vi "Object Items (poly).vi"   [LabVIEW 2019, in "JSONtext.lvlib"]
doc: "Find multiple Items in a JSON Object, by item names. Output items (as JSON) are in the same order as the supplied item names. If an item is not present, then the output for that item will be an empty string.\n\nThe location, in the input JSON, of the Object containing the items may be specified either by Offset or by a JSON Path (polymorphic input)."
uses:
  JSONtext.lvlib
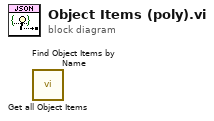
[diagram p0: block diagram]
diagram:
  n1 = call "Get all Object Items.vi"() -> ()  [unwired: 8 in, 4 out]
  n2 = call "Find Object Items by Name.vi"() -> ()  [unwired: 9 in, 3 out]
